vi "pattern_recognition.vi"(0 "read buffer in":string) -> (2 "read buffer out":string, 3 "Boolean":bool)   [LabVIEW 2016]
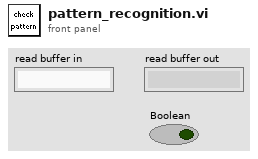
[diagram p1: front panel]
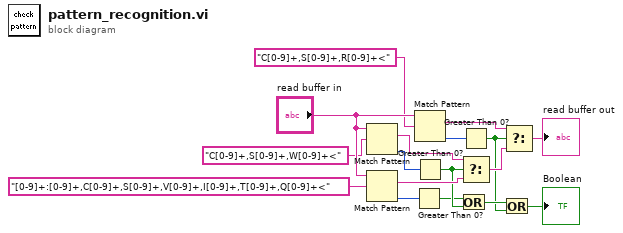
[diagram p0: block diagram]
diagram:
  n1 = Match Pattern(string="read buffer in", regular expression="C[0-9]+,S[0-9]+,W[0-9]+<") -> (match substring=w10:string, offset past match=w6:i32)  [unwired: 1 in, 2 out]
  n2 = Match Pattern(string="read buffer in", regular expression="[0-9]+:[0-9]+,C[0-9]+,S[0-9]+,V[0-9]+,I[0-9]+,T[0-9]+,Q[0-9]+<") -> (match substring=w9:string, offset past match=w2:i32)  [unwired: 1 in, 2 out]
  n3 = Greater Than 0?(x=w2) -> (x > 0?=w1:bool)
  n4 = Match Pattern(string="read buffer in", regular expression="C[0-9]+,S[0-9]+,R[0-9]+<") -> (match substring=w15:string, offset past match=w4:i32)  [unwired: 1 in, 2 out]
  n5 = Greater Than 0?(x=w6) -> (x > 0?=w5:bool)
  n6 = Or(x=w1, y=w5) -> (x .or. y?=w16:bool)
  n7 = Greater Than 0?(x=w4) -> (x > 0?=w3:bool)
  n8 = Select(t=w10, s=w5, f=w9) -> (s? t:f=w13:string)
  n9 = Or(x=w16, y=w3) -> (x .or. y?=→"Boolean":bool)
  n10 = Select(t=w15, s=w3, f=w13) -> (s? t:f=→"read buffer out":string)
